vi "Handle Data.vi"(8 "error in (no error)":errorcluster, 10 "Data":T1, 11 "LocalGraphBuffer in":refnum<class "LocalGraphBuffer.lvclass">) -> (0 "error out":errorcluster)   [LabVIEW 2020, in "VolatusGUIElements.lvlib" / "LocalGraphBuffer.lvclass"]
uses:
  LocalGraphBuffer.lvclass
  lv-vecto/Vecto/Subscribed Data.ctl
  LocalGraphBuffer.lvclass/LocalGraphBuffer.ctl
  lv-vecto/Vecto/Vecto.lvlib
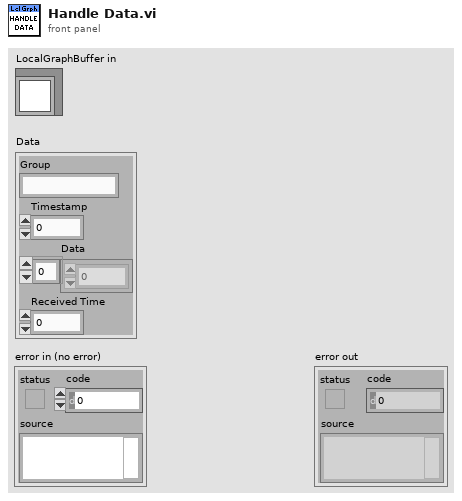
[diagram p1: front panel]
types:
  T1 = typedef "Vecto.lvlib/Subscribed Data.ctl" = cluster{"Group":string, "Timestamp":dbl, "Data":dbl[], "Received Time":dbl}
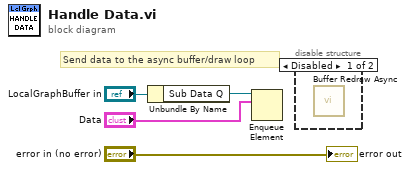
[diagram p0: block diagram]
diagram:
  # "Send data to the async buffer/draw loop"
  n1 = Unbundle By Name("LocalGraphBuffer in") -> ("Sub Data Q"=w2:refnum<queue>)
  n2 = Enqueue Element(queue=w2, element="Data") -> ()  [unwired: 2 in, 3 out]
  n3 = disable-structure shown="Disabled" {
    frame Disabled {
      n4 = call "Buffer Redraw Async.vi"() -> ()  [unwired: 12 in]
    }
    frame Enabled {
    }
  }
  "error out" <- "error in (no error)"
